vi "traj_generator.vi"(0 "v_max":dbl, 1 "a_max":dbl, 3 "p_f":dbl, 5 "v_f":dbl, 6 "trigger":bool, 7 "t":dbl) -> (14 "p":dbl format="%0.2f", 15 "v":dbl format="%0.2f", 16 "a":dbl)   [LabVIEW 2014]
doc: "Based on :\nTime-Optimal Online Trajectory Generator for Robotic Manipulators \nFransisco Ramos. et al.\n\nInputs:\na_max = maximum admissible acceleration\nv_max = maximum admissible speed\np_i = current position\np_f = target position\nv_i = current velocity\nv_f = target velocity\ntrigger = tell the algorithm to proceed\nThe trigger signal is a transition from 0 to 1 (edge triggered)\n\nOutputs:\na = acceleration trajectory\nv = velocitiy trajectory\np = position trajectory"
panel:
  out "is_triggered":bool
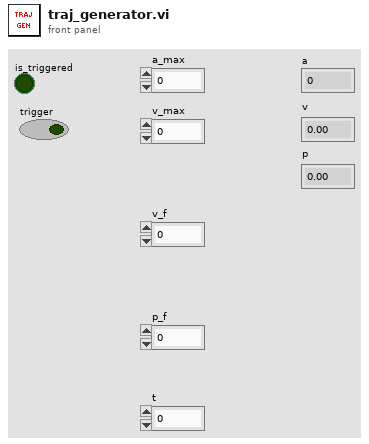
[diagram p1: front panel]
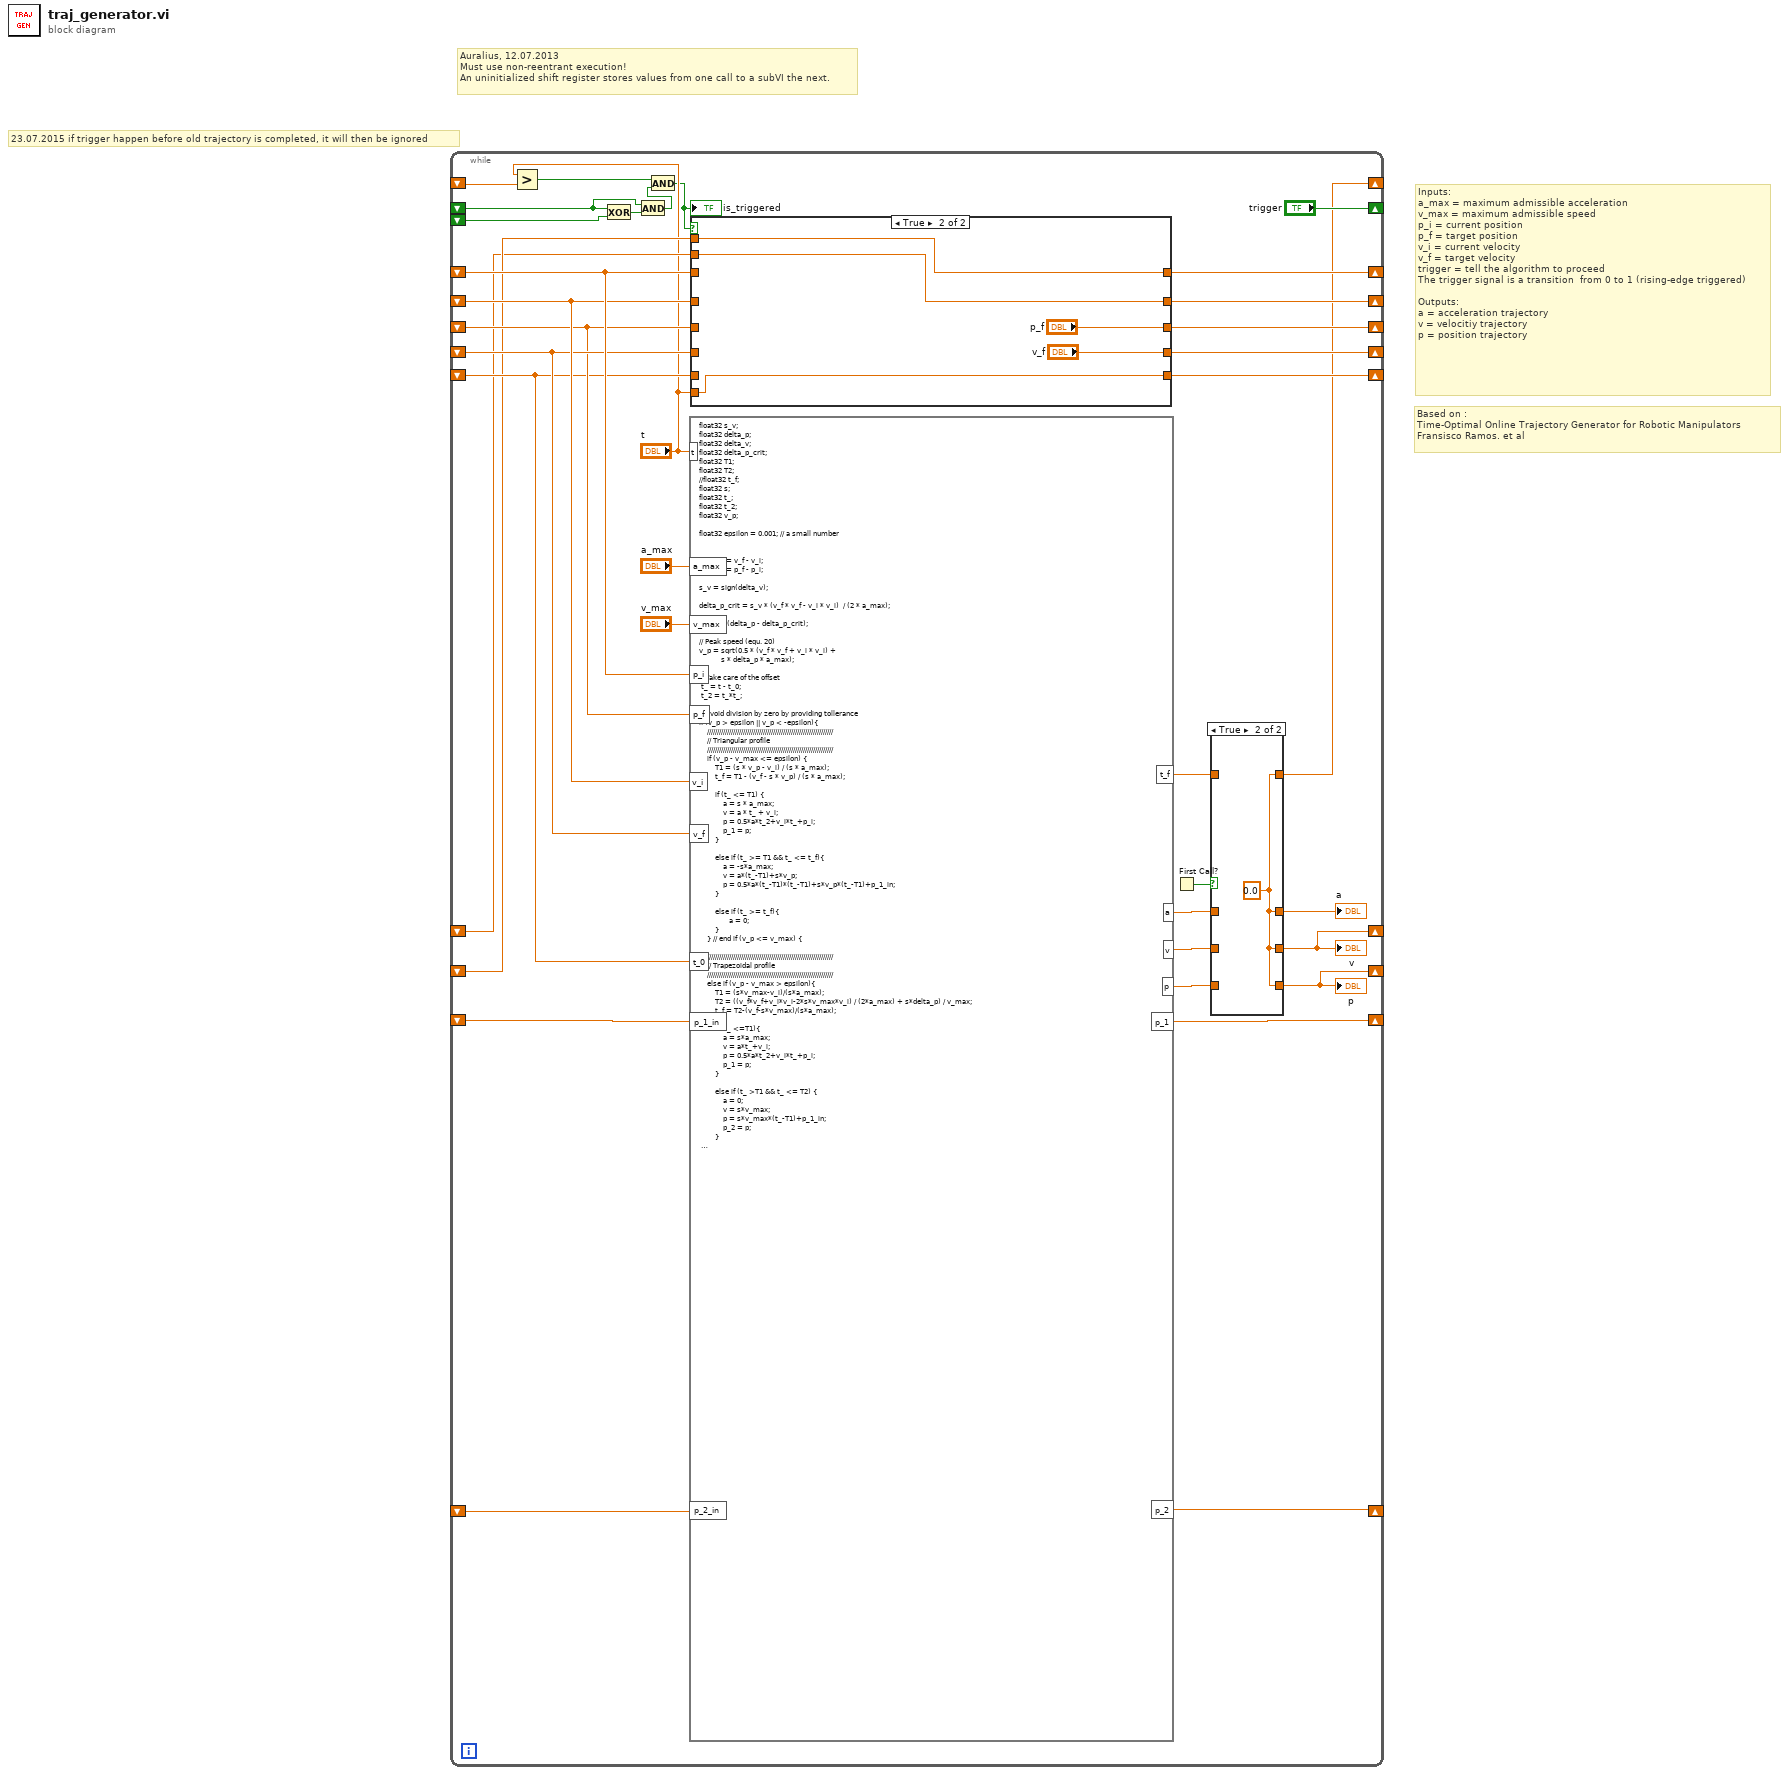
[diagram p0: block diagram]
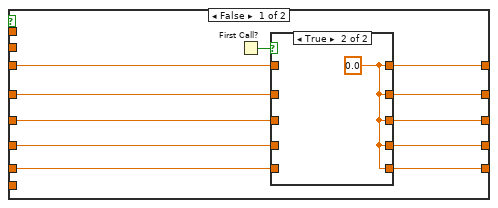
[diagram p3: hidden frame]
diagram:
  # "23.07.2015 if trigger happen before old trajectory is completed, it will then be ignored"
  # "Based on :\nTime-Optimal Online Trajectory Generator for Robotic Manipulators \nFransisco Ramos. et al"
  # "Inputs:\na_max = maximum admissible acceleration\nv_max = maximum admissible speed\np_i = current position\np_f = target position\nv_i = current velocity\nv_f = target velocity\ntrigger = tell the algorithm to proceed\nThe trigger signal is a transition  from 0 to 1 (rising-edge triggered)\n\nOutputs:\na = acceleration trajectory\nv = velocitiy trajectory\np = position trajectory"
  # "Auralius, 12.07.2013\nMust use non-reentrant execution!\nAn uninitialized shift register stores values from one call to a subVI the next."
  n1 = while {
    shift-right: ["trigger"] -> _
    shift-left: _ -> [w32]
    shift-left: _ -> [w33]
    shift-right: [w30] -> _
    shift-left: _ -> [w28]
    shift-right: [w29] -> _
    shift-left: _ -> [w27]
    shift-right: [w25] -> _
    shift-left: _ -> [w22]
    shift-right: [w24] -> _
    shift-left: _ -> [w23]
    shift-right: [w21] -> _
    shift-left: _ -> [w20]
    shift-right: [w16] -> _
    shift-left: _ -> [w17]
    shift-right: [w15] -> _
    shift-left: _ -> [w14]
    shift-right: [w11] -> _
    shift-left: _ -> [w10]
    shift-right: [w9] -> _
    shift-left: _ -> [w8]
    shift-right: [w2] -> _
    shift-left: _ -> [w7]
    stop <- FALSE continue-if-true
    n2 = Greater?(x="t", y=w7) -> (0:w5:bool)
    n3 = Exclusive Or(1:w33, 2:w32) -> (0:w31:bool)
    n4 = And(x=w32, y=w31) -> (x .and. y?=w4:bool)
    n5 = And(x=w5, y=w4) -> (x .and. y?=w3:bool)
    "is_triggered" <- w3
    n6 = formula code="float32 s_v;\nfloat32 delta_p;\nfloat32 delta_v;\nfloat32 delta_p_crit;\nfloat32 T1;\nfloat32 T2;\n//float32 t_f;\nfloat32 s;\nfloat32 t_;\nfloat32 t_2;\nfloat32 v_p;\n\nfloat32 epsilon = 0.001; // a small number\n\n\ndelta_v = v_f - v_i;\ndelta_p = p_f - p_i;\n\ns_v = sign(delta_v);\n\ndelta_p_crit = s_v * (v_f * v_f - v_i * v_i)  / (2 * a_max);\n\ns = sign(delta_p - delta_p_crit);\n\n// Peak speed (equ. 20)\nv_p = sqrt(0.5 * (v_f * v_f + v_i * v_i) + \n           s * delta_p * a_max);\n\n// Take care of the offset\n t_ = t - t_0;\n t_2 = t_*t_;\n\n// Avoid division by zero by providing tollerance          \nif (v_p > epsilon || v_p < -epsilon){\n    ///////////////////////////////////////////////////////////////\n    // Triangular profile\n    ///////////////////////////////////////////////////////////////\n    if (v_p - v_max <= epsilon) {\n        T1 = (s * v_p - v_i) / (s * a_max);\n        t_f = T1 - (v_f - s * v_p) / (s * a_max);\n\n        if (t_ <= T1) {\n            a = s * a_max;\n            v = a * t_ + v_i;\n            p = 0.5*a*t_2+v_i*t_+p_i;\n            p_1 = p;\n        } \n\n        else if (t_ >= T1 && t_ <= t_f){\n            a = -s*a_max;\n            v = a*(t_-T1)+s*v_p;\n            p = 0.5*a*(t_-T1)*(t_-T1)+s*v_p*(t_-T1)+p_1_in;\n        }\n\n        else if (t_ >= t_f){\n               a = 0;\n        }\n    } // end if (v_p <= v_max) {\n\n    ///////////////////////////////////////////////////////////////\n    // Trapezoidal profile\n    ///////////////////////////////////////////////////////////////\n    else if (v_p - v_max > epsilon){\n        T1 = (s*v_max-v_i)/(s*a_max);\n        T2 = ((v_f*v_f+v_i*v_i-2*s*v_max*v_i) / (2*a_max) + s*delta_p) / v_max;\n        t_f = T2-(v_f-s*v_max)/(s*a_max);\n\n        if (t_ <=T1){\n            a = s*a_max;\n            v = a*t_+v_i;\n            p = 0.5*a*t_2+v_i*t_+p_i; \n            p_1 = p;\n        }\n         \n        else if (t_ >T1 && t_ <= T2) {\n            a = 0;\n            v = s*v_max;\n            p = s*v_max*(t_-T1)+p_1_in;\n            p_2 = p;\n        }\n        \n        else if (t_>T2 && t_<=t_f){\n            a = -s*a_max;\n            v = a*(t_-T2)+s*v_max;\n            p = 0.5*a*(t_-T2)*(t_-T2)+s*v_max*(t_-T2)+p_2_in;\n        }\n\n        else if (t_ > t_f){\n               a = 0;\n        }\n    } // end else if (v_p > v_max){\n} \n\nelse{\n    a=0;\n    v=v_i;\n    p = p_i;\n}  \n///////////////////////////////////////////////////////////////"("a_max"="a_max", "v_max"="v_max", "v_i"=w27, "v_f"=w23, "p_i"=w28, "p_f"=w22, "t"="t", "t_0"=w20, "p_1_in"=w17, "p_2_in"=w14) -> ("a"=w26:dbl, "v"=w19:dbl, "p"=w18:dbl, "p_1"=w16:dbl, "p_2"=w15:dbl, "t_f"=w1:dbl)
    n7 = case shown="True" w3 {
      tunnel: [w44 w61] -> w30
      tunnel: [w46 w60] -> w29
      tunnel: w28 -> [w43 _]
      tunnel: w27 -> [w45 _]
      tunnel: [w48 "p_f"] -> w25
      tunnel: [w50 "v_f"] -> w24
      tunnel: w22 -> [w47 _]
      tunnel: w23 -> [w49 _]
      tunnel: [w52 w62] -> w21
      tunnel: w20 -> [w51 _]
      tunnel: "t" -> [_ w62]
      tunnel: w10 -> [_ w61]
      tunnel: w8 -> [_ w60]
      frame False {
        n8 = First Call?() -> (First Call?: T/F=w53:bool)
        n9 = case shown="True" w53 {
          tunnel: [w58 w59] -> w52
          tunnel: w51 -> [w58 _]
          tunnel: [w57 w59] -> w50
          tunnel: w49 -> [w57 _]
          tunnel: [w56 w59] -> w48
          tunnel: w47 -> [w56 _]
          tunnel: [w55 w59] -> w46
          tunnel: w45 -> [w55 _]
          tunnel: [w54 w59] -> w44
          tunnel: w43 -> [w54 _]
          frame False {
          }
          frame True {
            w59 = 0.0 ("p_i")
          }
        }
      }
      frame True {
      }
    }
    n10 = First Call?() -> (First Call?: T/F=w13:bool)
    n11 = case shown="True" w13 {
      tunnel: w26 -> [w41 _]
      tunnel: w19 -> [w40 _]
      tunnel: w18 -> [w39 _]
      tunnel: [w41 w42] -> w12
      tunnel: [w40 w42] -> w9
      tunnel: [w39 w42] -> w11
      tunnel: [w38 w42] -> w2
      tunnel: w1 -> [w38 _]
      frame False {
      }
      frame True {
        w42 = 0.0 ("a")
      }
    }
    "a" <- w12
    "v" <- w9
    "p" <- w11
  }
